vi "1L10_proba_1D-en-txt_1D.vi"(1 "proba num":dbl[](array[numeric])) -> (0 "proba txt":string[](array[string]))   [LabVIEW 2010, in "lv_01.lvlib"]
uses:
  lv_01.lvlib
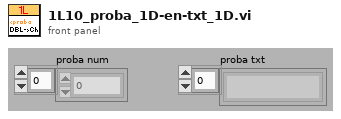
[diagram p1: front panel]
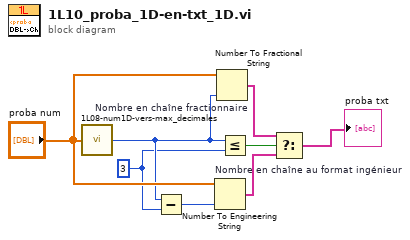
[diagram p0: block diagram]
diagram:
  w2 = 3 ("y")
  n1 = call "1L08-num1D-vers-max_decimales.vi"("num. déc. (1D)"="proba num") -> ("Max déc."=w3:i32)
  n2 = Subtract(x=w3, y=w2) -> (x-y=w1:i32)
  n3 = Number To Engineering String "Nombre en chaîne au format ingénieur"(2:w1, 4:"proba num") -> (0:w7:string[])  [unwired: 2 in]
  n4 = Number To Fractional String "Nombre en chaîne fractionnaire"(number="proba num", precision (6)=w3) -> (F-format string=w5:string[])  [unwired: 2 in]
  n5 = Less Or Equal?(x=w3, y=w2) -> (x <= y?=w4:bool)
  n6 = Select(t=w5, s=w4, f=w7) -> (s? t:f=→"proba txt":string[])
